vi "Builder.LoadedFromProject.vi"(8 "error in":errorcluster, 11 "App Refnum":refnum<vi>) -> (0 "error out":errorcluster, 1 "FilesInProject":path[](array[path]), 3 "ProjectPath":path)   [LabVIEW 2011]
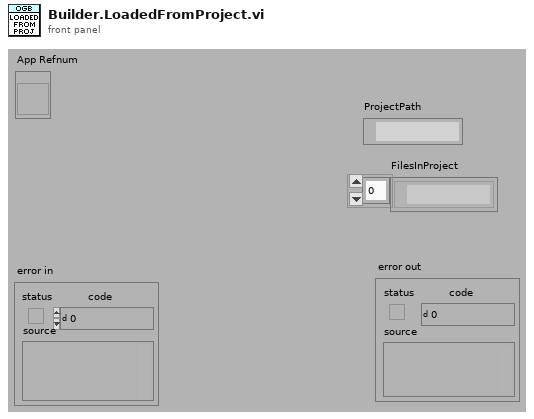
[diagram p1: front panel]
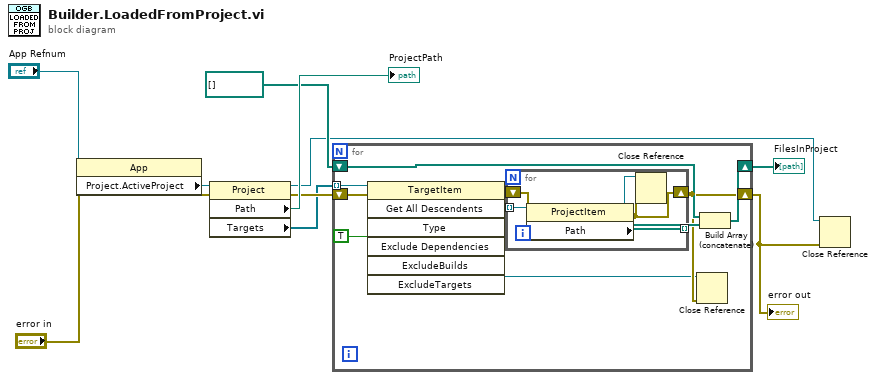
[diagram p0: block diagram]
diagram:
  n1 = property class="App"(reference="App Refnum", error in="error in") -> (error out=w8:errorcluster, "Project.ActiveProject"=w9:refnum<vi>)  [unwired: 1 out]
  n2 = property class="Project"(reference=w9, error in=w8) -> (reference out=w2:refnum<vi>, error out=w6:errorcluster, "Path"=→"ProjectPath":path, "Targets"=w5:refnum<vi>[])
  n3 = for {
    tunnel: w5 -> [w20] mode=indexing
    shift-right: [w13] -> w1
    shift-left: w6 -> [w21]
    shift-right: [w15] -> w3
    shift-left: path[] [] -> [w17]
    w14 = TRUE ("ExcludeDependencies")
    n4 = invoke class="TargetItem" method="Get All Descendents"(reference=w20, error in=w21, "Exclude Dependencies"=w14, "ExcludeBuilds"=w14, "ExcludeTargets"=w14) -> (reference out=w12:refnum<vi>, error out=w19:errorcluster, "All Descendents"=w18:refnum<vi>[])  [unwired: 2 in, 4 out]
    n5 = for {
      tunnel: w18 -> [w25] mode=indexing
      tunnel: [w24] -> w16 mode=indexing
      shift-right: [w23] -> w13
      shift-left: w19 -> [w26]
      n6 = property class="ProjectItem"(reference=w25, error in=w26) -> (reference out=w22:refnum<vi>, error out=w23:errorcluster, "Path"=w24:path)
      n7 = Close Reference(reference=w22, error in (no error)=w23) -> ()  [unwired: 1 out]
    }
    n8 = Close Reference(reference=w12, error in (no error)=w13) -> ()  [unwired: 1 out]
    n9 = Build Array (concatenate)(w17, w16) -> (w15:path[])
  }
  "error out" <- w1
  "FilesInProject" <- w3
  n10 = Close Reference(reference=w2, error in (no error)=w1) -> ()  [unwired: 1 out]
